vi "trapezoidal_teste.vi"() -> ()   [LabVIEW 2020]
uses:
  <vilib>/Analysis/NI_AALBase.lvlib
panel:
  in  "Amplitude":dbl(knob)=3.7755102040816326 scale=0.0..5.0
  in  "Wave Table":dbl[](array[numeric])=[0.0, 1.0, 4.0, 0.2, -0.9]
  in  "interpolation":i32(ring)=1 items=["none", "linear"]
  out "Waveform Pattern":dbl[](graph)
  in  "Frequency":dbl(knob)=2.01 step=1.0 scale=0.0..10.0
  in  "Stop":bool
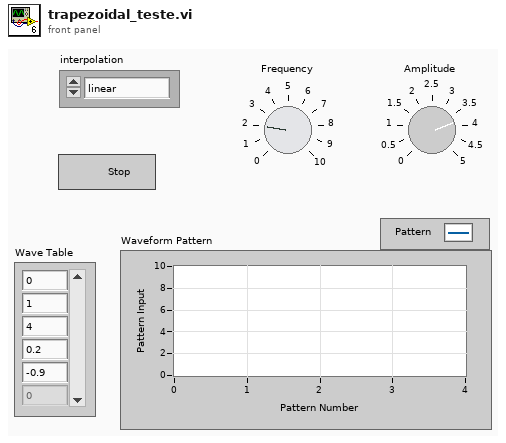
[diagram p1: front panel]
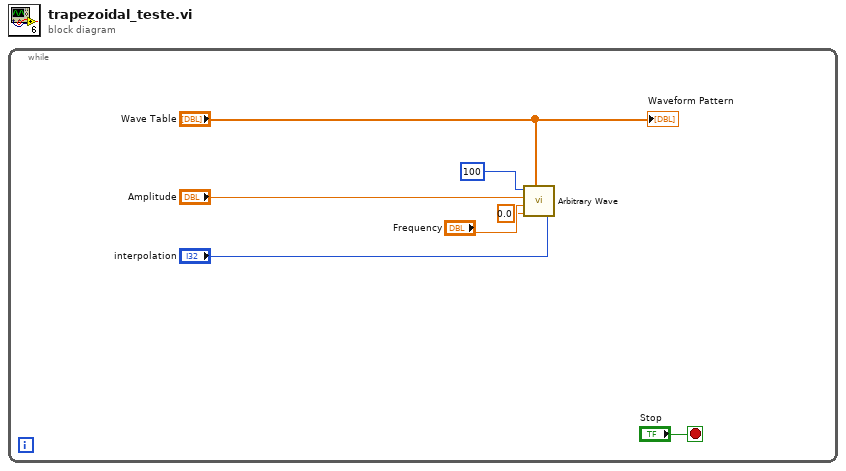
[diagram p0: block diagram]
diagram:
  n1 = while {
    stop <- "Stop" stop-if-true
    n2 = call <vilib>:"Arbitrary Wave.vi"("interpolation"="interpolation", "Wave Table"="Wave Table", "phase in"=0.0, "frequency"="Frequency", "amplitude"="Amplitude", "samples"=100) -> ()  [unwired: 1 in, 3 out]
    "Waveform Pattern" <- "Wave Table"
  }
